vi "Handle getAll.vi"(8 "error in (no error)":errorcluster, 11 "Inst.TSL210 in":refnum<class "Inst.TSL210.lvclass">) -> (0 "error out":errorcluster, 2 "getAll":variant, 3 "Inst.TSL210 out":refnum<class "Inst.TSL210.lvclass">)   [LabVIEW 2019, in "Inst.TSL210.lvclass"]
uses:
  Inst.TSL210.lvclass
  Typedefs/Inst.TSL210.getAll--Cluster.ctl
  Inst.TSL210.lvclass/Inst.TSL210.ctl
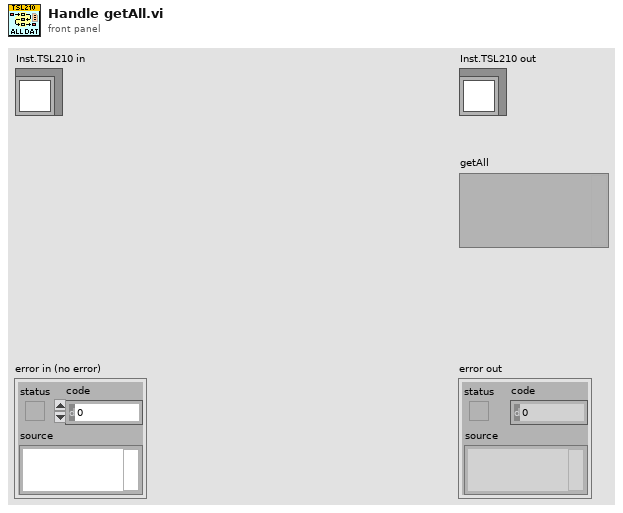
[diagram p1: front panel]
types:
  T1 = typedef "Inst.TSL210.lvclass/Inst.TSL210.getAll--Cluster.ctl" = cluster{"Wavelength (nm)":dbl, "Power (mW)":dbl, "Status: LD":bool, "Status: COH":bool, "Status: TempError":bool, "Status: CurrentLimit":bool, "Status: SystemBusy":bool, "Status: ATT":bool, "Status: ACC":bool, "Status: FT":bool}
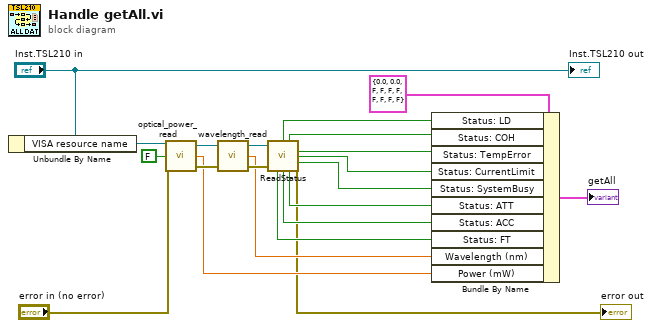
[diagram p0: block diagram]
diagram:
  n1 = Unbundle By Name("Inst.TSL210 in") -> ("VISA resource name"=w8:refnum<visa-resource-name>)
  n2 = call "optical_power_read.vi"("error in (no error)"="error in (no error)", "unit"=FALSE, "VISA session (for class)"=w8) -> ("error out"=w5:errorcluster, "optical power"=w2:dbl, "dup VISA session"=w7:refnum<visa-resource-name>)
  n3 = call "wavelength_read.vi"("VISA session (for class)"=w7, "error in (no error)"=w5) -> ("dup VISA session"=w6:refnum<visa-resource-name>, "wavelength in nm (numerical output)"=w3:ext, "error out"=w4:errorcluster)
  n4 = call "ReadStatus.vi"("VISA session"=w6, "error in (no error)"=w4) -> ("LD ON"=w18:bool, "COH"=w17:bool, "Temp. Err."=w16:bool, "Current Limit"=w15:bool, "Busy"=w14:bool, "FT"=w11:bool, "ACC"=w12:bool, "ATT"=w13:bool, "error out"=→"error out":errorcluster)  [unwired: 3 in, 2 out]
  n5 = Bundle By Name(cluster=T1 {"Wavelength (nm)"=0.0, "Power (mW)"=0.0, "Status: LD"=FALSE, "Status: COH"=FALSE, "Status: TempError"=FALSE, "Status: CurrentLimit"=FALSE, "Status: SystemBusy"=FALSE, "Status: ATT"=FALSE, "Status: ACC"=FALSE, "Status: FT"=FALSE} ("getAll"), "Status: LD"=w18, "Status: COH"=w17, "Status: TempError"=w16, "Status: CurrentLimit"=w15, "Status: SystemBusy"=w14, "Status: ATT"=w13, "Status: ACC"=w12, "Status: FT"=w11, "Wavelength (nm)"=w3, "Power (mW)"=w2) -> (→"getAll":T1)
  "Inst.TSL210 out" <- "Inst.TSL210 in"
